vi "Shooter.vi"(9 "Aquisition + Scoring 2":T1={"Aquisition MotorControlDeviceRef"={"DeviceStatus"={"status"=FALSE, "code"=0, "source"=""}, "Type"=enum."PWM", "PWM"={"PWM Channel"=enum."Invalid", "DeadBand"={"Name"="", "maxPositivePwm"=0, "minPositivePwm"=0, "centerPwm"=0, "maxNegativePwm"=0, "minNegativePwm"=0, "angularRange"=0}}, "CAN"={"Device Number"=0, "Control Mode"=enum."Percent VBus", "Semaphore"=refnum, "Max Vout"=12.0, "TalonSRX Control Mode"=enum."Percent VBus"}, "Invert"=FALSE}, "Scoring 1 MotorControlDeviceRef"={"DeviceStatus"={"status"=FALSE, "code"=0, "source"=""}, "Type"=enum."PWM", "PWM"={"PWM Channel"=enum."Invalid", "DeadBand"={"Name"="", "maxPositivePwm"=0, "minPositivePwm"=0, "centerPwm"=0, "maxNegativePwm"=0, "minNegativePwm"=0, "angularRange"=0}}, "CAN"={"Device Number"=0, "Control Mode"=enum."Percent VBus", "Semaphore"=refnum, "Max Vout"=12.0, "TalonSRX Control Mode"=enum."Percent VBus"}, "Invert"=FALSE}, "Scoring 2 MotorControlDeviceRef"={"DeviceStatus"={"status"=FALSE, "code"=0, "source"=""}, "Type"=enum."PWM", "PWM"={"PWM Channel"=enum."Invalid", "DeadBand"={"Name"="", "maxPositivePwm"=0, "minPositivePwm"=0, "centerPwm"=0, "maxNegativePwm"=0, "minNegativePwm"=0, "angularRange"=0}}, "CAN"={"Device Number"=0, "Control Mode"=enum."Percent VBus", "Semaphore"=refnum, "Max Vout"=12.0, "TalonSRX Control Mode"=enum."Percent VBus"}, "Invert"=FALSE}, "Roller MotorControlDeviceRef"={"DeviceStatus"={"status"=FALSE, "code"=0, "source"=""}, "Type"=enum."PWM", "PWM"={"PWM Channel"=enum."Invalid", "DeadBand"={"Name"="", "maxPositivePwm"=0, "minPositivePwm"=0, "centerPwm"=0, "maxNegativePwm"=0, "minNegativePwm"=0, "angularRange"=0}}, "CAN"={"Device Number"=0, "Control Mode"=enum."Percent VBus", "Semaphore"=refnum, "Max Vout"=12.0, "TalonSRX Control Mode"=enum."Percent VBus"}, "Invert"=FALSE}}) -> (3 "Aquisition + Scoring 3":T1={"Aquisition MotorControlDeviceRef"={"DeviceStatus"={"status"=FALSE, "code"=0, "source"=""}, "Type"=enum."PWM", "PWM"={"PWM Channel"=enum."Invalid", "DeadBand"={"Name"="", "maxPositivePwm"=0, "minPositivePwm"=0, "centerPwm"=0, "maxNegativePwm"=0, "minNegativePwm"=0, "angularRange"=0}}, "CAN"={"Device Number"=0, "Control Mode"=enum."Percent VBus", "Semaphore"=refnum, "Max Vout"=12.0, "TalonSRX Control Mode"=enum."Percent VBus"}, "Invert"=FALSE}, "Scoring 1 MotorControlDeviceRef"={"DeviceStatus"={"status"=FALSE, "code"=0, "source"=""}, "Type"=enum."PWM", "PWM"={"PWM Channel"=enum."Invalid", "DeadBand"={"Name"="", "maxPositivePwm"=0, "minPositivePwm"=0, "centerPwm"=0, "maxNegativePwm"=0, "minNegativePwm"=0, "angularRange"=0}}, "CAN"={"Device Number"=0, "Control Mode"=enum."Percent VBus", "Semaphore"=refnum, "Max Vout"=12.0, "TalonSRX Control Mode"=enum."Percent VBus"}, "Invert"=FALSE}, "Scoring 2 MotorControlDeviceRef"={"DeviceStatus"={"status"=FALSE, "code"=0, "source"=""}, "Type"=enum."PWM", "PWM"={"PWM Channel"=enum."Invalid", "DeadBand"={"Name"="", "maxPositivePwm"=0, "minPositivePwm"=0, "centerPwm"=0, "maxNegativePwm"=0, "minNegativePwm"=0, "angularRange"=0}}, "CAN"={"Device Number"=0, "Control Mode"=enum."Percent VBus", "Semaphore"=refnum, "Max Vout"=12.0, "TalonSRX Control Mode"=enum."Percent VBus"}, "Invert"=FALSE}, "Roller MotorControlDeviceRef"={"DeviceStatus"={"status"=FALSE, "code"=0, "source"=""}, "Type"=enum."PWM", "PWM"={"PWM Channel"=enum."Invalid", "DeadBand"={"Name"="", "maxPositivePwm"=0, "minPositivePwm"=0, "centerPwm"=0, "maxNegativePwm"=0, "minNegativePwm"=0, "angularRange"=0}}, "CAN"={"Device Number"=0, "Control Mode"=enum."Percent VBus", "Semaphore"=refnum, "Max Vout"=12.0, "TalonSRX Control Mode"=enum."Percent VBus"}, "Invert"=FALSE}})   [LabVIEW 2015]
uses:
  Robot Values.vi
  <vilib>/Rock Robotics/WPI/MotorControl/WPI_MotorControlDeviceRef.ctl
  <vilib>/Rock Robotics/WPI/CAN/Jaguar/SubVIs/WPI_CANJaguar_ControlMode.ctl
  <vilib>/Rock Robotics/WPI/CAN/TalonSRX/WPI_CANTalonSRX_APIControlMode.ctl
  <vilib>/Rock Robotics/SystemInterfaces/DIO/FPGA_DIOPWMChannel.ctl
  <vilib>/Rock Robotics/WPI/PWM/WPI_PWMDeadband.ctl
  <vilib>/Rock Robotics/WPI/MotorControl/WPI_MotorControlType.ctl
  Acquisition & Scoring.ctl
panel:
  in  "Shoot?":bool
  in  "Acquire?":bool
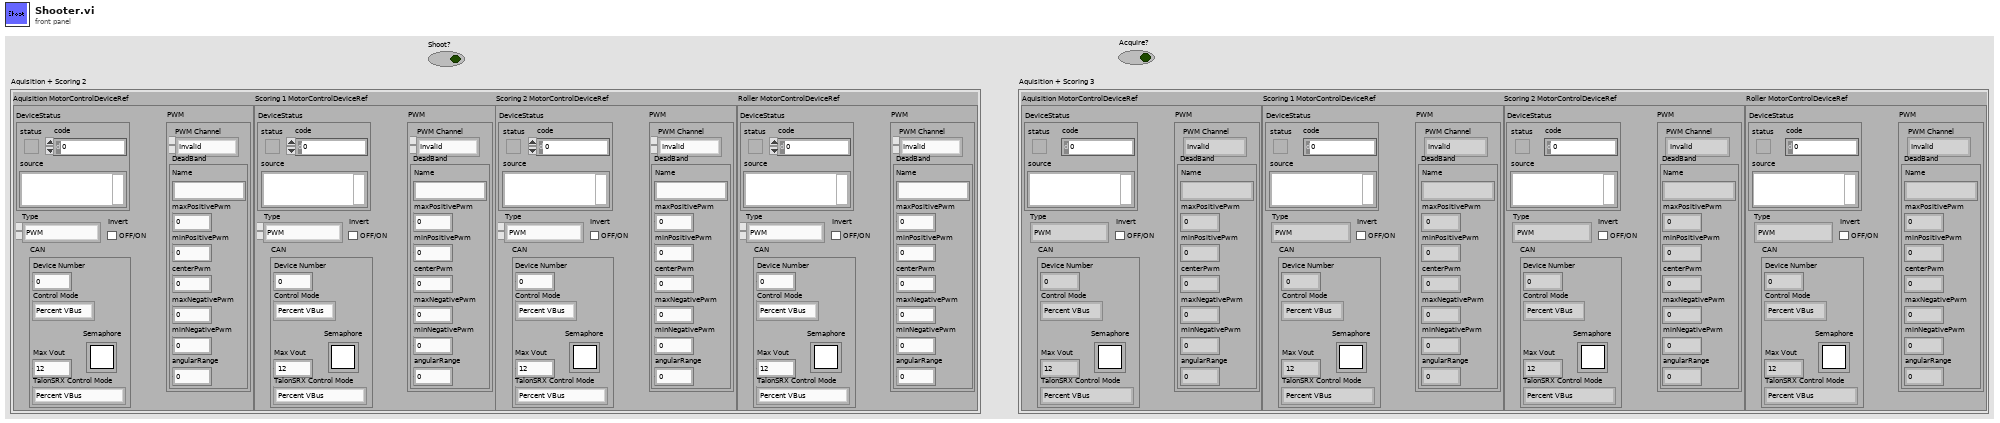
[diagram p1: front panel]
types:
  T1 = typedef "Acquisition & Scoring.ctl" = cluster{"Aquisition MotorControlDeviceRef":T2, "Scoring 1 MotorControlDeviceRef":T2, "Scoring 2 MotorControlDeviceRef":T2, "Roller MotorControlDeviceRef":T2}
  T2 = typedef "WPI_MotorControlDeviceRef.ctl" = cluster{"DeviceStatus":errorcluster, "Type":T3, "PWM":cluster{"PWM Channel":T4, "DeadBand":T5}, "CAN":cluster{"Device Number":u8, "Control Mode":T6, "Semaphore":T7, "Max Vout":dbl, "TalonSRX Control Mode":T8}, "Invert":bool}
  T3 = typedef "WPI_MotorControlType.ctl" = enum16{"PWM", "CAN", "CANTalonSRX"}
  T4 = typedef "FPGA_DIOPWMChannel.ctl" = enum8{"PWM 0", "PWM 1", "PWM 2", "PWM 3", "PWM 4", "PWM 5", "PWM 6", "PWM 7", "PWM 8", "PWM 9", "PWM MXP 0", "PWM MXP 1", "PWM MXP 2", "PWM MXP 3", "PWM MXP 4", "PWM MXP 5", "PWM MXP 6", "PWM MXP 7", "PWM MXP 8", "PWM MXP 9", "Invalid"}
  T5 = typedef "WPI_PWMDeadband.ctl" = cluster{"Name":string, "maxPositivePwm":i32, "minPositivePwm":i32, "centerPwm":i32, "maxNegativePwm":i32, "minNegativePwm":i32, "angularRange":u16}
  T6 = typedef "WPI_CANJaguar_ControlMode.ctl" = enum8{"Percent VBus", "Current", "Speed", "Position", "Voltage"}
  T7 = typedef "Semaphore RefNum" = refnum<k1>
  T8 = typedef "WPI_CANTalonSRX_APIControlMode.ctl" = enum8{"Percent VBus", "Speed", "Position", "Slave", "Unchanged / Invalid", "Voltage Compensation", "Current", "Motion Profile"}
  T9 = typedef "Drive Values.ctl" = cluster{"Drive Motors":cluster{"Left Motor Value":dbl, "Right Motor Value":dbl, "Left Motor Encoder":dbl, "Right Motor Encoder":dbl, "High/Low Gear":bool, "PTO":bool}, "Sensors":cluster{"Gyro Angle":dbl, "Hanging Limit":bool, "Photoeye":bool, "Ultrasonic Range":dbl, "Shooter Speed Encoder":dbl}, "Arms":cluster{"Arm Position":dbl, "Left Arm Encoder":dbl, "Right Arm Encoder":dbl, "Left Arm Lower Limit":bool, "Right Arm Lower Limit":bool}, "Acquisition and Scoring":cluster{"Acquiring?":bool, "Rotation Counter":dbl}}
  T10 = typedef "WPI_AnalogChannelDevRef.ctl" = cluster{"DevStatus":errorcluster, "Analog Channel":T11}
  T11 = typedef "FPGA_AIChannel.ctl" = enum8{"AI 0", "AI 1", "AI 2", "AI 3", "AI MXP 0", "AI MXP 1", "AI MXP 2", "AI MXP 3", "Invalid"}
  T12 = cluster{"Aquisition MotorControlDeviceRef":T2, "Scoring 1 MotorControlDeviceRef":T2, "Scoring 2 MotorControlDeviceRef":T2, "Roller MotorControlDeviceRef":T2, "Shooter Encoder AIDeviceRef":T10}
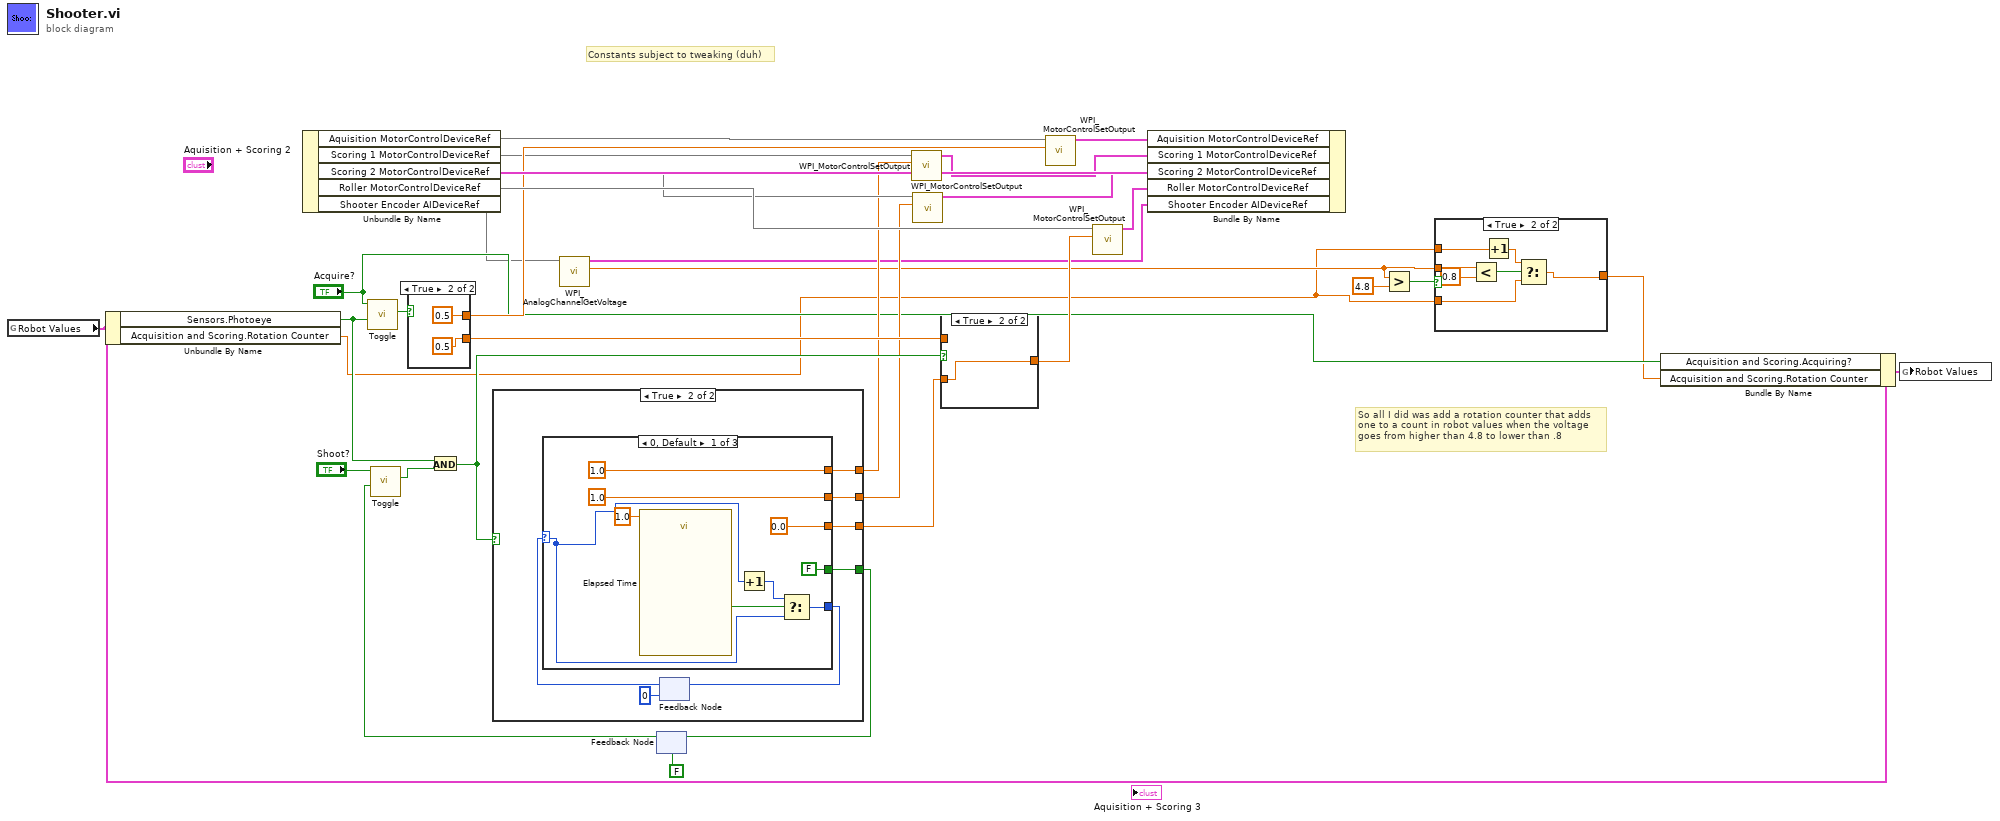
[diagram p0: block diagram]
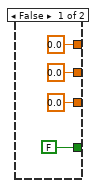
[diagram p3: hidden frame]
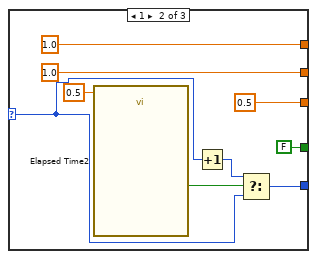
[diagram p4: hidden frame]
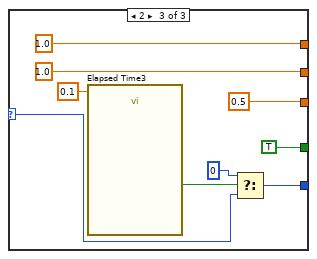
[diagram p5: hidden frame]
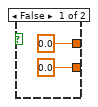
[diagram p7: hidden frame]
diagram:
  # "So all I did was add a rotation counter that adds \none to a count in robot values when the voltage \ngoes from higher than 4.8 to lower than .8"
  # "Constants subject to tweaking (duh)"
  n1 = global read "Robot Values.vi" "Robot Values"() -> (w10:T9)
  n2 = Unbundle By Name(w10) -> ("Sensors.Photoeye"=w9:bool, "Acquisition and Scoring.Rotation Counter"=w1:dbl)
  n3 = Unbundle By Name() -> (w29:T12, "Aquisition MotorControlDeviceRef"=w33, "Scoring 1 MotorControlDeviceRef"=w26, "Scoring 2 MotorControlDeviceRef"=w25, "Roller MotorControlDeviceRef"=w31, "Shooter Encoder AIDeviceRef"=w7)
  n4 = call "Toggle.vi"("Internal Toggle"=w9, "User Toggle"="Acquire?") -> ("True/False"=w28:bool)  [unwired: 9 in]
  n5 = case shown="True" w28 {
    tunnel: [0.0 0.5] -> w27
    tunnel: [0.0 0.5] -> w20
    frame False {
    }
    frame True {
    }
  }
  n6 = call <vilib>:"WPI_AnalogChannelGetVoltage.vi"("AIDeviceRef"=w7) -> ("Voltage"=w3:dbl, "AIDeviceRef"=w6:T10)  [unwired: 8 in, 1 out]
  n7 = feedback #1(FALSE) -> (w17:bool)
  n8 = call "Toggle.vi"("Internal Toggle"=w17, "User Toggle"="Shoot?") -> ("True/False"=w21:bool)  [unwired: 9 in]
  n9 = And(x=w9, y=w21) -> (x .and. y?=w16:bool)
  n10 = case shown="True" w16 {
    tunnel: [0.0 w48] -> w15
    tunnel: [0.0 w47] -> w14
    tunnel: [0.0 w44] -> w13
    tunnel: [FALSE w43] -> w18
    frame False {
    }
    frame True {
      n11 = feedback #2(0 ("t")) -> (w45:i32)
      n12 = case shown="0, Default" w45 {
        selector: w45 -> [w53 w59 w69]
        tunnel: [1.0 1.0 1.0] -> w48
        tunnel: [1.0 1.0 1.0] -> w47
        tunnel: [w51 w60 w70] -> w46
        tunnel: [0.0 0.5 0.5] -> w44
        tunnel: [FALSE FALSE TRUE] -> w43
        frame 0, Default {
          n13 = call "Elapsed Time"("Time Target (s)"=1.0) -> ("Time has Elapsed"=w54:bool)  [unwired: 11 in, 7 out]
          n14 = Increment(x=w53) -> (x+1=w52:i32)
          n15 = Select(t=w52, s=w54, f=w53) -> (s? t:f=w51:i32)
        }
        frame 1 {
          n16 = call "Elapsed Time2"("Time Target (s)"=0.5) -> ("Time has Elapsed"=w65:bool)  [unwired: 11 in, 7 out]
          n17 = Increment(x=w59) -> (x+1=w64:i32)
          n18 = Select(t=w64, s=w65, f=w59) -> (s? t:f=w60:i32)
        }
        frame 2 {
          n19 = call "Elapsed Time3"("Time Target (s)"=0.1) -> ("Time has Elapsed"=w74:bool)  [unwired: 11 in, 7 out]
          n20 = Select(t=0, s=w74, f=w69) -> (s? t:f=w70:i32)
        }
      }
      n21 = feedback-in #2(w46) -> ()
    }
  }
  n22 = feedback-in #1(w18) -> ()
  n23 = call <vilib>:"WPI_MotorControlSetOutput.vi"("Output"=w15, "MotorControlDevRef"=w26) -> ("MotorControlDevRef"=w24:T2)  [unwired: 7 in, 2 out]
  n24 = call <vilib>:"WPI_MotorControlSetOutput.vi"("Output"=w14, "MotorControlDevRef"=w25) -> ("MotorControlDevRef"=w23:T2)  [unwired: 7 in, 2 out]
  n25 = case shown="True" w16 {
    tunnel: w20 -> [w76 _]
    tunnel: [w76 w77] -> w19
    tunnel: w13 -> [_ w77]
    frame False {
    }
    frame True {
    }
  }
  n26 = call <vilib>:"WPI_MotorControlSetOutput.vi"("Output"=w27, "MotorControlDevRef"=w33) -> ("MotorControlDevRef"=w32:T2)  [unwired: 7 in, 2 out]
  n27 = call <vilib>:"WPI_MotorControlSetOutput.vi"("Output"=w19, "MotorControlDevRef"=w31) -> ("MotorControlDevRef"=w30:T2)  [unwired: 7 in, 2 out]
  n28 = Bundle By Name(cluster=w29, "Aquisition MotorControlDeviceRef"=w32, "Scoring 1 MotorControlDeviceRef"=w24, "Scoring 2 MotorControlDeviceRef"=w23, "Roller MotorControlDeviceRef"=w30, "Shooter Encoder AIDeviceRef"=w6) -> ()  [unwired: 1 out]
  n29 = Greater?(x=w3, y=4.8) -> (0:w4:bool)
  n30 = case shown="True" w4 {
    tunnel: w3 -> [_ w85]
    tunnel: [w78 w82] -> w2
    tunnel: w1 -> [_ w80]
    tunnel: w1 -> [w78 w79]
    frame False {
    }
    frame True {
      n31 = Less?(x=w85, y=0.8) -> (x < y?=w83:bool)
      n32 = Increment(x=w80) -> (x+1=w81:dbl)
      n33 = Select(t=w81, s=w83, f=w79) -> (s? t:f=w82:dbl)
    }
  }
  n34 = Bundle By Name(cluster=w10, "Acquisition and Scoring.Acquiring?"="Acquire?", "Acquisition and Scoring.Rotation Counter"=w2) -> (w11:T9)
  n35 = global write "Robot Values.vi" "Robot Values"(w11) -> ()
